vi "CMD Update DUT Parameters.vi"(8 "error in (no error)":errorcluster, 10 "vData":variant, 11 "DAQ in":refnum<class "DAQ.lvclass">) -> (0 "error out":errorcluster, 3 "DAQ out":refnum<class "DAQ.lvclass">)   [LabVIEW 2017]
uses:
  DAQ.lvclass
  DataTypes/AsyncMsg_DAQ--enum.ctl
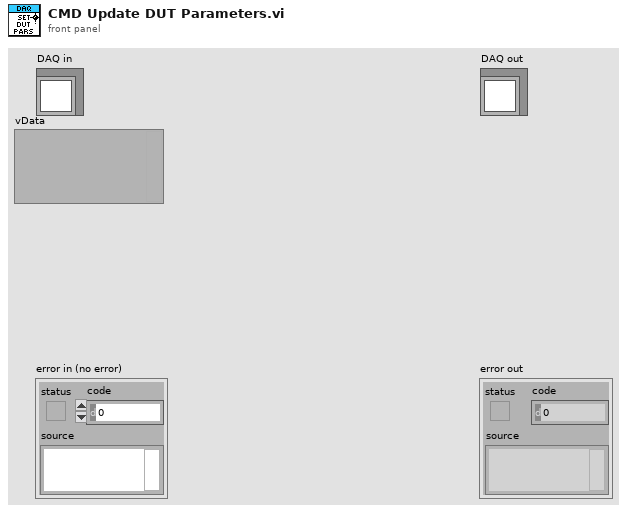
[diagram p1: front panel]
types:
  T1 = typedef "DAQ.lvclass/AsyncMsg_DAQ--enum.ctl" = enum16{"StartDAQ", "StopDAQ", "OpenTDMS", "CloseTDMS", "StartTDMSLogging", "StopTDMSLogging", "Open&StartTDMSLogging", "Stop&CloseTDMSLogging", "CfgDAQ", "UpdateDUTParameters", "UpdateSeqPath"}
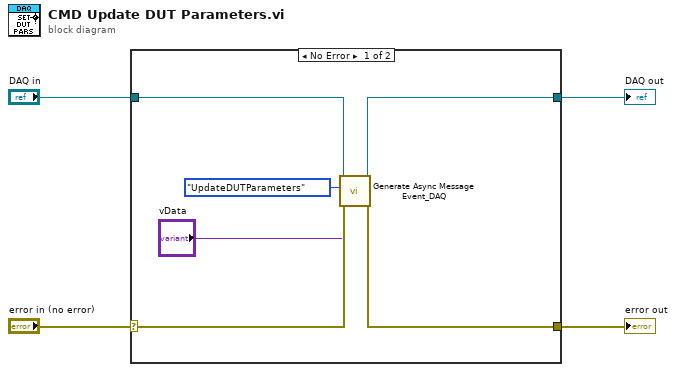
[diagram p0: block diagram]
diagram:
  n1 = case shown="No Error" "error in (no error)" {
    selector: "error in (no error)" -> [w10 w12]
    tunnel: [w9 w12] -> w3
    tunnel: [w7 w11] -> w1
    tunnel: "DAQ in" -> [w8 w11]
    frame No Error {
      n2 = call "Generate Async Message Event_DAQ.vi"("error in (no error)"=w10, "vData"="vData", "AsyncMsg"=AsyncMsg_DAQ--enum."UpdateDUTParameters", "DAQ"=w8) -> ("error out"=w9:errorcluster, "DAQ out"=w7:refnum<class "DAQ.lvclass">)  [unwired: 6 in]
    }
    frame Error {
    }
  }
  "error out" <- w3
  "DAQ out" <- w1
